vi "ApproachingPart_WangYunong.vi"() -> ()   [LabVIEW 2014]
uses:
  <vilib>/Instr/_visa.llb/VISA Configure Serial Port (Instr).vi
panel:
  in  "ZFinalHeldPos um":dbl
  out "Not Ascend of RZ":bool
  out "AfterMax":dbl
  out "RefCurr":dbl format="%#_13g"
  out "RoughZMov":dbl(graph)
  out "RZPos?":string
  out "CURR":string
  out "POS":dbl(graph)
  out "step":i32
  out "Err1":string
  in  "stop":bool
  out "Curr to Step":dbl(graph)
  out "Curr to Pos":cluster{dbl[], dbl[]}(graph)
  out "ZPos?":dbl
  out "RoughZERR?":string
  out "PIZERR?":string
  in  "ConstantCurrPIZ":refnum<visa-resource-name>="COM1"
  in  "Amp":refnum<visa-resource-name>="GPIB0::8::INSTR"
  in  "Moving":refnum<visa-resource-name>="COM6"
  out "OutLeak":string
  in  "ZApproachingThresholdDecline %":dbl format="%#_13g"
  in  "ZApproachPerStep um":dbl format="%#_13g"
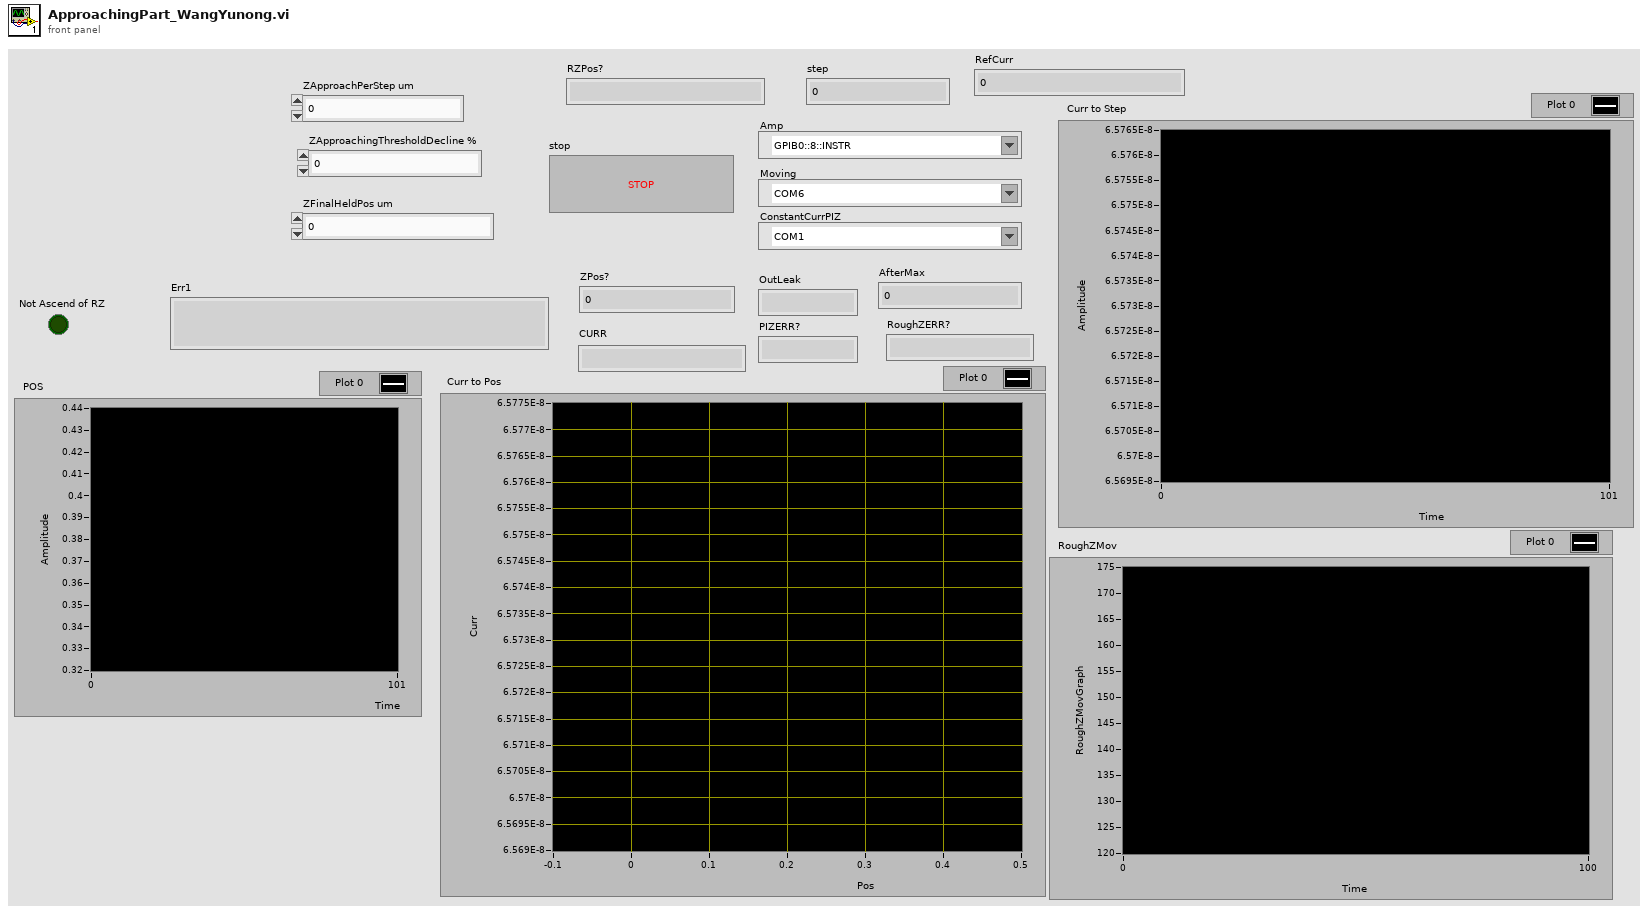
[diagram p1: front panel]
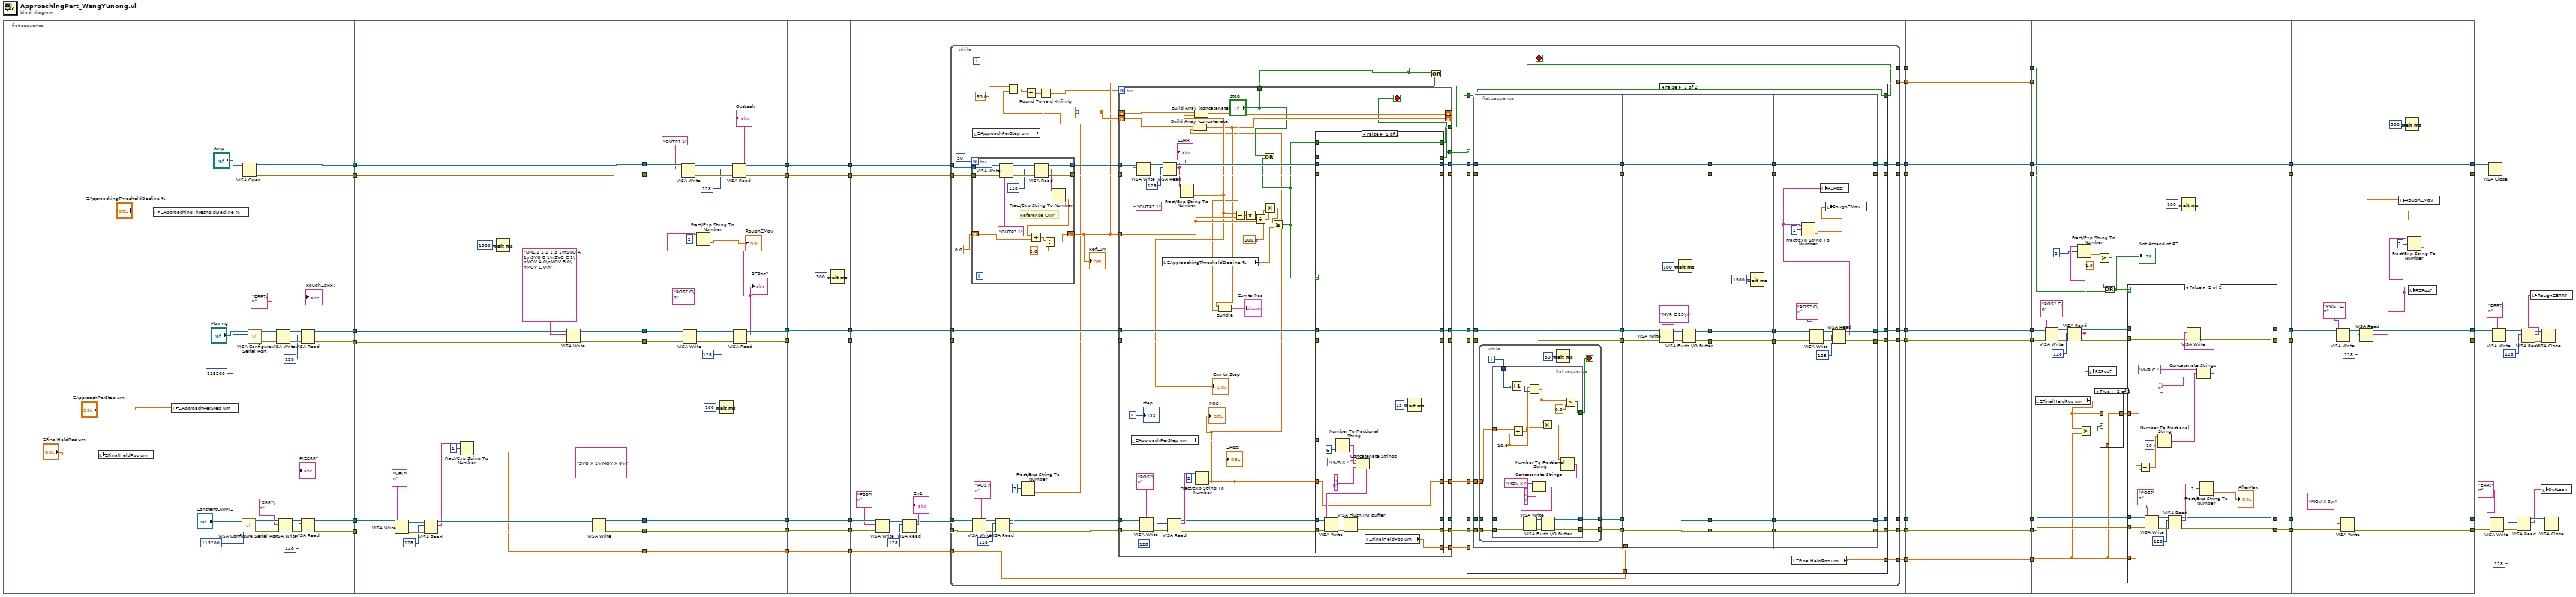
[diagram p0: block diagram]
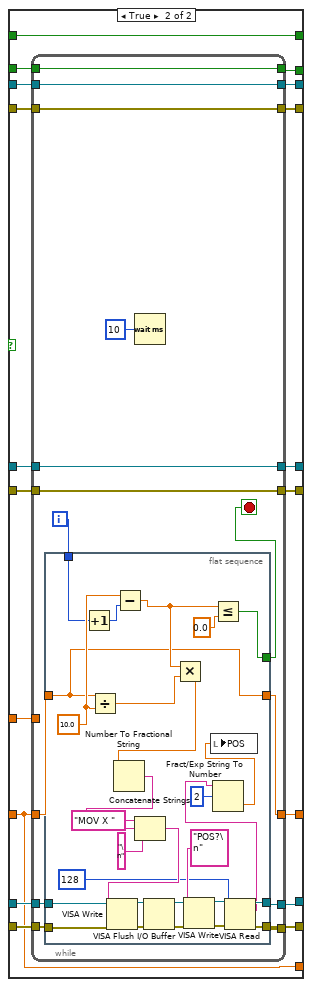
[diagram p3: hidden frame]
diagram:
  n1 = flat-sequence {
    tunnel: [w88] -> w53
    tunnel: [w87] -> w52
    tunnel: [w82] -> w51
    tunnel: [w81] -> w50
    tunnel: [w77] -> w49
    tunnel: [w76] -> w48
    tunnel: [w121] -> w71
    tunnel: [w120] -> w70
    tunnel: [w104] -> w69
    tunnel: [w103] -> w68
    tunnel: [w118] -> w67
    tunnel: [w117] -> w66
    tunnel: w53 -> [w104]
    tunnel: w52 -> [w103]
    tunnel: w51 -> [w106]
    tunnel: w50 -> [w105]
    tunnel: w49 -> [w111]
    tunnel: w48 -> [w110]
    tunnel: [w100] -> w47
    tunnel: w71 -> [w131]
    tunnel: w70 -> [w130]
    tunnel: w69 -> [w145]
    tunnel: w68 -> [w144]
    tunnel: [w129] -> w60
    tunnel: [w128] -> w61
    tunnel: [w143] -> w62
    tunnel: [w142] -> w63
    tunnel: w67 -> [w123]
    tunnel: w66 -> [w122]
    tunnel: [w123] -> w64
    tunnel: [w122] -> w65
    tunnel: w47 -> [w135]
    tunnel: [w135] -> w45
    tunnel: w65 -> [w153]
    tunnel: [w153] -> w59
    tunnel: w64 -> [w152]
    tunnel: [w152] -> w58
    tunnel: w63 -> [w151]
    tunnel: [w151] -> w57
    tunnel: w62 -> [w150]
    tunnel: [w150] -> w56
    tunnel: w61 -> [w149]
    tunnel: [w149] -> w55
    tunnel: w60 -> [w148]
    tunnel: [w148] -> w54
    tunnel: [w146] -> w46
    tunnel: w45 -> [w146]
    tunnel: w59 -> [w159]
    tunnel: w58 -> [w160]
    tunnel: w57 -> [w173]
    tunnel: w56 -> [w174]
    tunnel: w55 -> [w175]
    tunnel: w54 -> [w176]
    tunnel: [w172] -> w18
    tunnel: [w171] -> w16
    tunnel: [w170] -> w14
    tunnel: [w169] -> w12
    tunnel: [w168] -> w10
    tunnel: [w167] -> w8
    tunnel: [w166] -> w6
    tunnel: w46 -> [w165]
    tunnel: [w154] -> w4
    tunnel: [w155] -> w2
    tunnel: w18 -> [w489]
    tunnel: [w489] -> w17
    tunnel: w16 -> [w488]
    tunnel: [w488] -> w15
    tunnel: w14 -> [w487]
    tunnel: [w487] -> w13
    tunnel: w12 -> [w486]
    tunnel: [w486] -> w11
    tunnel: w10 -> [w485]
    tunnel: [w485] -> w9
    tunnel: w8 -> [w484]
    tunnel: [w484] -> w7
    tunnel: w6 -> [w483]
    tunnel: [w483] -> w5
    tunnel: w4 -> [w482]
    tunnel: [w482] -> w3
    tunnel: w2 -> [w481]
    tunnel: [w481] -> w1
    tunnel: w17 -> [w517]
    tunnel: w15 -> [w516]
    tunnel: w13 -> [w504]
    tunnel: w11 -> [w503]
    tunnel: w9 -> [w514]
    tunnel: w7 -> [w513]
    tunnel: w5 -> [_]
    tunnel: w3 -> [w490]
    tunnel: [w510] -> w44
    tunnel: [w509] -> w43
    tunnel: [w512] -> w42
    tunnel: [w511] -> w41
    tunnel: [w517] -> w40
    tunnel: [w516] -> w39
    tunnel: w1 -> [w495]
    tunnel: w44 -> [w560]
    tunnel: w43 -> [w559]
    tunnel: w42 -> [w551]
    tunnel: w41 -> [w550]
    tunnel: w40 -> [w554]
    tunnel: w39 -> [w553]
    tunnel: [w558] -> w31
    tunnel: [w557] -> w30
    tunnel: [w548] -> w27
    tunnel: [w547] -> w26
    tunnel: [w554] -> w29
    tunnel: [w553] -> w28
    frame #0 {
      n2 = local write "ZFinalHeldPos um"("ZFinalHeldPos um") -> ()
      n3 = local write "ZApproachingThresholdDecline %"("ZApproachingThresholdDecline %") -> ()
      n4 = local write "ZApproachPerStep um"("ZApproachPerStep um") -> ()
      n5 = call-poly "VISA Configure Serial Port"("VISA resource name"="ConstantCurrPIZ", "baud rate (9600)"=u32 115200) -> ("VISA resource name out"=w95:refnum<visa-resource-name>, "error out"=w94:errorcluster)  [unwired: 12 in]
      n6 = VISA Open(VISA resource name="Amp") -> (VISA resource name=w88:refnum<visa-resource-name>, error out=w87:errorcluster)  [unwired: 4 in]
      n7 = call-poly "VISA Configure Serial Port"("VISA resource name"="Moving", "baud rate (9600)"=u32 115200) -> ("VISA resource name out"=w92:refnum<visa-resource-name>, "error out"=w91:errorcluster)  [unwired: 12 in]
      n8 = VISA Write(VISA resource name=w92, write buffer="ERR?\n", error in (no error)=w91) -> (VISA resource name out=w83:refnum<visa-resource-name>, error out=w84:errorcluster)  [unwired: 1 out]
      n9 = VISA Write(VISA resource name=w95, write buffer="ERR?\n", error in (no error)=w94) -> (VISA resource name out=w79:refnum<visa-resource-name>, error out=w78:errorcluster)  [unwired: 1 out]
      n10 = VISA Read(VISA resource name=w83, byte count=u32 128, error in (no error)=w84) -> (VISA resource name out=w82:refnum<visa-resource-name>, read buffer=→"RoughZERR?":string, error out=w81:errorcluster)  [unwired: 1 out]
      n11 = VISA Read(VISA resource name=w79, byte count=u32 128, error in (no error)=w78) -> (VISA resource name out=w77:refnum<visa-resource-name>, read buffer=→"PIZERR?":string, error out=w76:errorcluster)  [unwired: 1 out]
    }
    frame #1 {
      n12 = VISA Write(VISA resource name=w111, write buffer="VEL?\n", error in (no error)=w110) -> (VISA resource name out=w114:refnum<visa-resource-name>, error out=w113:errorcluster)  [unwired: 1 out]
      n13 = VISA Read(VISA resource name=w114, byte count=u32 128, error in (no error)=w113) -> (VISA resource name out=w109:refnum<visa-resource-name>, read buffer=w102:string, error out=w108:errorcluster)  [unwired: 1 out]
      n14 = Fract/Exp String To Number(string=w102, offset=1) -> (number=w100:dbl)  [unwired: 2 in, 1 out]
      n15 = Wait (ms)(milliseconds to wait=u32 1500) -> ()  [unwired: 1 out]
      n16 = VISA Write(VISA resource name=w106, write buffer="ONL 1 1 2 1 3 1\nSVO A 1\nSVO B 1\nSVO C 1\nMOV A 0\nMOV B 0\nMOV C 0\n", error in (no error)=w105) -> (VISA resource name out=w121:refnum<visa-resource-name>, error out=w120:errorcluster)  [unwired: 1 out]
      n17 = VISA Write(VISA resource name=w109, write buffer="SVO X 1\nMOV X 0\n", error in (no error)=w108) -> (VISA resource name out=w118:refnum<visa-resource-name>, error out=w117:errorcluster)  [unwired: 1 out]
    }
    frame #2 {
      n18 = VISA Write(VISA resource name=w145, write buffer="OUTP? 1", error in (no error)=w144) -> (VISA resource name out=w141:refnum<visa-resource-name>, error out=w140:errorcluster)  [unwired: 1 out]
      n19 = VISA Write(VISA resource name=w131, write buffer="POS? C\n", error in (no error)=w130) -> (VISA resource name out=w134:refnum<visa-resource-name>, error out=w133:errorcluster)  [unwired: 1 out]
      n20 = Wait (ms)(milliseconds to wait=u32 100) -> ()  [unwired: 1 out]
      n21 = VISA Read(VISA resource name=w141, byte count=u32 128, error in (no error)=w140) -> (VISA resource name out=w143:refnum<visa-resource-name>, read buffer=→"OutLeak":string, error out=w142:errorcluster)  [unwired: 1 out]
      n22 = VISA Read(VISA resource name=w134, byte count=u32 128, error in (no error)=w133) -> (VISA resource name out=w129:refnum<visa-resource-name>, read buffer=w124:string, error out=w128:errorcluster)  [unwired: 1 out]
      "RZPos?" <- w124
      n23 = Fract/Exp String To Number(string=w124, offset=2) -> (number=→"RoughZMov":dbl)  [unwired: 2 in, 1 out]
    }
    frame #3 {
      n24 = Wait (ms)(milliseconds to wait=u32 300) -> ()  [unwired: 1 out]
    }
    frame #4 {
      n25 = VISA Write(VISA resource name=w160, write buffer="ERR?\n", error in (no error)=w159) -> (VISA resource name out=w164:refnum<visa-resource-name>, error out=w163:errorcluster)  [unwired: 1 out]
      n26 = VISA Read(VISA resource name=w164, byte count=u32 128, error in (no error)=w163) -> (VISA resource name out=w158:refnum<visa-resource-name>, read buffer=→"Err1":string, error out=w157:errorcluster)  [unwired: 1 out]
      n27 = while {
        tunnel: w176 -> [w218]
        tunnel: w175 -> [w216]
        tunnel: w174 -> [w223]
        tunnel: w173 -> [w222]
        tunnel: w158 -> [w186]
        tunnel: w157 -> [w185]
        tunnel: [w210] -> w170
        tunnel: [w209] -> w169
        tunnel: [w208] -> w172
        tunnel: [w207] -> w171
        tunnel: [w206] -> w168
        tunnel: [w205] -> w167
        tunnel: [w200] -> w166
        tunnel: w165 -> [w204]
        tunnel: [w198] -> w155
        tunnel: [w197] -> w154
        stop <- w194 stop-if-true
        w203 = dbl[] []
        n28 = for {
          N: 50 -> [_]
          tunnel: w223 -> [w232]
          tunnel: w222 -> [w231]
          tunnel: [w230] -> w220
          tunnel: [w229] -> w219
          shift-right: [w224] -> w200
          shift-left: 0.0 -> [w227]
          # "Reference Curr"
          n29 = VISA Write(VISA resource name=w232, write buffer="OUTP? 1", error in (no error)=w231) -> (VISA resource name out=w237:refnum<visa-resource-name>, error out=w236:errorcluster)  [unwired: 1 out]
          n30 = VISA Read(VISA resource name=w237, byte count=u32 128, error in (no error)=w236) -> (VISA resource name out=w230:refnum<visa-resource-name>, read buffer=w233:string, error out=w229:errorcluster)  [unwired: 1 out]
          n31 = Fract/Exp String To Number(string=w233) -> (number=w228:dbl)  [unwired: 3 in, 1 out]
          n32 = Add(x=w228, y=w227) -> (x+y=w226:dbl)
          n33 = Divide(x=w226, y=2.0) -> (x/y=w224:dbl)
        }
        "RefCurr" <- w200
        n34 = local read "ZApproachPerStep um"() -> (w178:dbl)
        n35 = VISA Write(VISA resource name=w186, write buffer="POS?\n", error in (no error)=w185) -> (VISA resource name out=w192:refnum<visa-resource-name>, error out=w191:errorcluster)  [unwired: 1 out]
        n36 = VISA Read(VISA resource name=w192, byte count=u32 128, error in (no error)=w191) -> (VISA resource name out=w184:refnum<visa-resource-name>, read buffer=w188:string, error out=w183:errorcluster)  [unwired: 1 out]
        n37 = Fract/Exp String To Number(string=w188, offset=2) -> (number=w177:dbl)  [unwired: 2 in, 1 out]
        n38 = Subtract(x=30.0, y=w177) -> (x-y=w181:dbl)
        n39 = Divide(x=w181, y=w178) -> (x/y=w180:dbl)
        n40 = Round Toward -Infinity(1:w180) -> (0:w179:dbl)
        n41 = for {
          N: w179 -> [_]
          tunnel: w184 -> [w377]
          tunnel: w183 -> [w376]
          tunnel: w200 -> [w391]
          tunnel: w220 -> [w395]
          tunnel: w219 -> [w394]
          tunnel: [w387] -> w212
          tunnel: [w386] -> w211
          tunnel: w218 -> [w385]
          tunnel: [w384] -> w217
          tunnel: w216 -> [w383]
          tunnel: [w382] -> w215
          tunnel: [w380] -> w214
          tunnel: [w379] -> w213
          tunnel: [w378] -> w202
          tunnel: [w369] -> w199
          shift-right: [w365] -> _
          shift-left: w203 -> [w368]
          shift-right: [w364] -> _
          shift-left: w203 -> [w367]
          tunnel: ["stop"] -> w198
          tunnel: [w351] -> w196
          tunnel: [w350] -> w193
          i -> [w358]
          stop <- w350 stop-if-true
          n42 = local read "ZApproachPerStep um"() -> (w381:dbl)
          n43 = VISA Write(VISA resource name=w395, write buffer="OUTP? 1", error in (no error)=w394) -> (VISA resource name out=w398:refnum<visa-resource-name>, error out=w397:errorcluster)  [unwired: 1 out]
          n44 = VISA Write(VISA resource name=w377, write buffer="POS?\n", error in (no error)=w376) -> (VISA resource name out=w375:refnum<visa-resource-name>, error out=w374:errorcluster)  [unwired: 1 out]
          n45 = local read "ZApproachingThresholdDecline %"() -> (w390:dbl)
          n46 = VISA Read(VISA resource name=w398, byte count=u32 128, error in (no error)=w397) -> (VISA resource name out=w389:refnum<visa-resource-name>, read buffer=w352:string, error out=w388:errorcluster)  [unwired: 1 out]
          "CURR" <- w352
          n47 = VISA Read(VISA resource name=w375, byte count=u32 128, error in (no error)=w374) -> (VISA resource name out=w360:refnum<visa-resource-name>, read buffer=w371:string, error out=w359:errorcluster)  [unwired: 1 out]
          n48 = Fract/Exp String To Number(string=w352) -> (number=w366:dbl)  [unwired: 3 in, 1 out]
          "Curr to Step" <- w366
          n49 = Build Array (concatenate)(w368, w366) -> (w365:dbl[])
          n50 = Fract/Exp String To Number(string=w371, offset=2) -> (number=w357:dbl)  [unwired: 2 in, 1 out]
          "ZPos?" <- w357
          "POS" <- w357
          n51 = Build Array (concatenate)(w367, w357) -> (w364:dbl[])
          n52 = Bundle(w364, w365) -> (→"Curr to Pos":cluster{dbl[], dbl[]})  [unwired: 1 in]
          n53 = Subtract(x=w366, y=w391) -> (x-y=w393:dbl)
          n54 = Absolute Value(x=w393) -> (abs(x)=w392:dbl)
          n55 = Divide(x=w392, y=w391) -> (x/y=w356:dbl)
          n56 = Multiply(x=w356, y=100.0) -> (x*y=w354:dbl)
          n57 = Greater Or Equal?(x=w354, y=w390) -> (x >= y?=w361:bool)
          n58 = Or(x="stop", y=w361) -> (x .or. y?=w353:bool)
          n59 = case shown="False" w361 {
            tunnel: w389 -> [w420 w431]
            tunnel: w388 -> [w419 w429]
            tunnel: [w420 w432] -> w387
            tunnel: [w419 w430] -> w386
            tunnel: w385 -> [w418 w427]
            tunnel: [w418 w428] -> w384
            tunnel: w383 -> [w417 w425]
            tunnel: [w417 w426] -> w382
            tunnel: w360 -> [w416 w437]
            tunnel: w359 -> [w415 w436]
            tunnel: w381 -> [w406 w433]
            tunnel: [w410 w435] -> w380
            tunnel: [w409 w434] -> w379
            tunnel: [w403 w438] -> w378
            tunnel: w361 -> [w403 w438]
            tunnel: w357 -> [w402 w421]
            tunnel: [w402 w424] -> w369
            tunnel: w353 -> [w401 w423]
            tunnel: [w401 w422] -> w350
            tunnel: [w400 w421] -> w351
            frame False {
              n60 = Number To Fractional String(number=w406, precision (6)=i16 6) -> (F-format string=w414:string)  [unwired: 2 in]
              n61 = Concatenate Strings("MVR X ", w414, "\n") -> (w411:string)
              n62 = VISA Write(VISA resource name=w416, write buffer=w411, error in (no error)=w415) -> (VISA resource name out=w408:refnum<visa-resource-name>, error out=w407:errorcluster)  [unwired: 1 out]
              n63 = VISA Flush I/O Buffer(VISA resource name=w408, error in (no error)=w407) -> (VISA resource name out=w410:refnum<visa-resource-name>, error out=w409:errorcluster)  [unwired: 1 in]
              n64 = local read "ZFinalHeldPos um"() -> (w400:dbl)
              n65 = Wait (ms)(milliseconds to wait=u32 15) -> ()  [unwired: 1 out]
            }
            frame True {
              n66 = while {
                tunnel: w437 -> [w446]
                tunnel: w436 -> [w445]
                tunnel: w421 -> [w444]
                tunnel: [w448] -> w435
                tunnel: [w447] -> w434
                tunnel: w433 -> [_]
                tunnel: [w452] -> w432
                tunnel: w431 -> [w452]
                tunnel: [w451] -> w430
                tunnel: w429 -> [w451]
                tunnel: [w450] -> w428
                tunnel: w427 -> [w450]
                tunnel: [w449] -> w426
                tunnel: w425 -> [w449]
                tunnel: [w441] -> w424
                tunnel: w423 -> [w439]
                tunnel: [w439] -> w422
                i -> [w443]
                stop <- w442 stop-if-true
                n67 = flat-sequence {
                  tunnel: w443 -> [w458]
                  tunnel: w446 -> [w478]
                  tunnel: w445 -> [w477]
                  tunnel: [w467] -> w448
                  tunnel: [w466] -> w447
                  tunnel: [w461] -> w442
                  tunnel: w444 -> [w455]
                  tunnel: [w455] -> w441
                  frame #0 {
                    w460 = 10.0
                    n68 = Increment(x=w458) -> (x+1=w459:i32)
                    n69 = Divide(x=w455, y=w460) -> (x/y=w454:dbl)
                    n70 = Subtract(x=w460, y=w459) -> (x-y=w456:dbl)
                    n71 = Multiply(x=w456, y=w454) -> (x*y=w453:dbl)
                    n72 = Number To Fractional String(number=w453) -> (F-format string=w476:string)  [unwired: 3 in]
                    n73 = Concatenate Strings("MOV X " ("string"), w476, "\n" ("string")) -> (w473:string)
                    n74 = VISA Write(VISA resource name=w478, write buffer=w473, error in (no error)=w477) -> (VISA resource name out=w480:refnum<visa-resource-name>, error out=w479:errorcluster)  [unwired: 1 out]
                    n75 = VISA Flush I/O Buffer(VISA resource name=w480, error in (no error)=w479) -> (VISA resource name out=w472:refnum<visa-resource-name>, error out=w471:errorcluster)  [unwired: 1 in]
                    n76 = VISA Write(VISA resource name=w472, write buffer="POS?\n", error in (no error)=w471) -> (VISA resource name out=w469:refnum<visa-resource-name>, error out=w468:errorcluster)  [unwired: 1 out]
                    n77 = Less Or Equal?(x=w456, y=0.0) -> (x <= y?=w461:bool)
                    n78 = VISA Read(VISA resource name=w469, byte count=u32 128, error in (no error)=w468) -> (VISA resource name out=w467:refnum<visa-resource-name>, read buffer=w463:string, error out=w466:errorcluster)  [unwired: 1 out]
                    n79 = Fract/Exp String To Number(string=w463, offset=2) -> (number=w462:dbl)  [unwired: 2 in, 1 out]
                    n80 = local write "POS"(w462) -> ()
                  }
                }
                n81 = Wait (ms)(milliseconds to wait=u32 10) -> ()  [unwired: 1 out]
              }
            }
          }
          "step" <- w358
        }
        n82 = Or(x=w198, y=w202) -> (x .or. y?=w195:bool)
        n83 = case shown="False" w193 {
          tunnel: w217 -> [w267 w349]
          tunnel: w215 -> [w266 w348]
          tunnel: w214 -> [w265 w345]
          tunnel: w213 -> [w264 w344]
          tunnel: w212 -> [w271 w347]
          tunnel: w211 -> [w269 w346]
          tunnel: [w263 w349] -> w210
          tunnel: [w262 w348] -> w209
          tunnel: [w270 w347] -> w208
          tunnel: [w268 w346] -> w207
          tunnel: [w261 w345] -> w206
          tunnel: [w260 w344] -> w205
          tunnel: w204 -> [w259 _]
          tunnel: w199 -> [w240 _]
          tunnel: [w238 w343] -> w197
          tunnel: w196 -> [_ w343]
          tunnel: w195 -> [w239 w342]
          tunnel: [w239 w342] -> w194
          frame False {
            n84 = flat-sequence {
              tunnel: w271 -> [w277]
              tunnel: w269 -> [w278]
              tunnel: w267 -> [w279]
              tunnel: w266 -> [w280]
              tunnel: w265 -> [w276]
              tunnel: w264 -> [w275]
              tunnel: [w273] -> w246
              tunnel: [w274] -> w245
              tunnel: [w280] -> w244
              tunnel: [w279] -> w243
              tunnel: [w278] -> w242
              tunnel: [w277] -> w241
              tunnel: w240 -> [w272]
              tunnel: [w319] -> w258
              tunnel: [w318] -> w256
              tunnel: [w310] -> w254
              tunnel: [w309] -> w252
              tunnel: [w312] -> w250
              tunnel: [w311] -> w248
              tunnel: w259 -> [_]
              tunnel: w246 -> [w309]
              tunnel: w245 -> [w310]
              tunnel: w244 -> [w314]
              tunnel: w243 -> [w315]
              tunnel: w242 -> [w318]
              tunnel: w241 -> [w319]
              tunnel: w258 -> [w326]
              tunnel: [w326] -> w257
              tunnel: w256 -> [w325]
              tunnel: [w325] -> w255
              tunnel: w254 -> [w324]
              tunnel: [w324] -> w253
              tunnel: w252 -> [w323]
              tunnel: [w323] -> w251
              tunnel: w250 -> [w322]
              tunnel: [w322] -> w249
              tunnel: w248 -> [w321]
              tunnel: [w321] -> w247
              tunnel: [w340] -> w268
              tunnel: [w341] -> w270
              tunnel: w257 -> [w341]
              tunnel: w255 -> [w340]
              tunnel: w253 -> [w339]
              tunnel: w251 -> [w338]
              tunnel: w249 -> [w333]
              tunnel: w247 -> [w332]
              tunnel: [w331] -> w263
              tunnel: [w330] -> w262
              tunnel: [w339] -> w261
              tunnel: [w338] -> w260
              frame #0 {
                n85 = while {
                  tunnel: w276 -> [w288]
                  tunnel: w275 -> [w287]
                  tunnel: [w286] -> w274
                  tunnel: [w285] -> w273
                  tunnel: w272 -> [w282]
                  i -> [w284]
                  stop <- w283 stop-if-true
                  n86 = flat-sequence {
                    tunnel: w284 -> [w297]
                    tunnel: w288 -> [w305]
                    tunnel: w287 -> [w304]
                    tunnel: [w303] -> w286
                    tunnel: [w302] -> w285
                    tunnel: [w290] -> w283
                    tunnel: w282 -> [w295]
                    frame #0 {
                      w294 = 10.0 ("y")
                      n87 = Increment(x=w297) -> (x+1=w296:i32)
                      n88 = Divide(x=w295, y=w294) -> (x/y=w293:dbl)
                      n89 = Subtract(x=w294, y=w296) -> (x-y=w291:dbl)
                      n90 = Multiply(x=w291, y=w293) -> (x*y=w289:dbl)
                      n91 = Number To Fractional String(number=w289) -> (F-format string=w301:string)  [unwired: 3 in]
                      n92 = Concatenate Strings("MOV X " ("string"), w301, "\n" ("string")) -> (w298:string)
                      n93 = VISA Write(VISA resource name=w305, write buffer=w298, error in (no error)=w304) -> (VISA resource name out=w307:refnum<visa-resource-name>, error out=w306:errorcluster)  [unwired: 1 out]
                      n94 = VISA Flush I/O Buffer(VISA resource name=w307, error in (no error)=w306) -> (VISA resource name out=w303:refnum<visa-resource-name>, error out=w302:errorcluster)  [unwired: 1 in]
                      n95 = Less Or Equal?(x=w291, y=0.0) -> (x <= y?=w290:bool)
                    }
                  }
                  n96 = Wait (ms)(milliseconds to wait=u32 30) -> ()  [unwired: 1 out]
                }
              }
              frame #1 {
                n97 = VISA Write(VISA resource name=w315, write buffer="MVR C 25\n", error in (no error)=w314) -> (VISA resource name out=w317:refnum<visa-resource-name>, error out=w316:errorcluster)  [unwired: 1 out]
                n98 = Wait (ms)(milliseconds to wait=u32 100) -> ()  [unwired: 1 out]
                n99 = VISA Flush I/O Buffer(VISA resource name=w317, error in (no error)=w316) -> (VISA resource name out=w312:refnum<visa-resource-name>, error out=w311:errorcluster)  [unwired: 1 in]
              }
              frame #2 {
                n100 = Wait (ms)(milliseconds to wait=u32 1500) -> ()  [unwired: 1 out]
              }
              frame #3 {
                n101 = VISA Write(VISA resource name=w333, write buffer="POS? C\n", error in (no error)=w332) -> (VISA resource name out=w336:refnum<visa-resource-name>, error out=w335:errorcluster)  [unwired: 1 out]
                n102 = VISA Read(VISA resource name=w336, byte count=u32 128, error in (no error)=w335) -> (VISA resource name out=w331:refnum<visa-resource-name>, read buffer=w329:string, error out=w330:errorcluster)  [unwired: 1 out]
                n103 = Fract/Exp String To Number(string=w329, offset=2) -> (number=w327:dbl)  [unwired: 2 in, 1 out]
                n104 = local write "RZPos?"(w329) -> ()
                n105 = local write "RoughZMov"(w327) -> ()
              }
            }
            n106 = local read "ZFinalHeldPos um"() -> (w238:dbl)
          }
          frame True {
          }
        }
      }
    }
    frame #5 {
    }
    frame #6 {
      n107 = local read "ZFinalHeldPos um"() -> (w492:dbl)
      n108 = VISA Write(VISA resource name=w504, write buffer="POS? C\n", error in (no error)=w503) -> (VISA resource name out=w507:refnum<visa-resource-name>, error out=w506:errorcluster)  [unwired: 1 out]
      n109 = VISA Read(VISA resource name=w507, byte count=u32 128, error in (no error)=w506) -> (VISA resource name out=w502:refnum<visa-resource-name>, read buffer=w500:string, error out=w501:errorcluster)  [unwired: 1 out]
      n110 = Fract/Exp String To Number(string=w500, offset=2) -> (number=w498:dbl)  [unwired: 2 in, 1 out]
      n111 = Greater?(x=w492, y=w490) -> (0:w493:bool)
      n112 = local write "RZPos?"(w500) -> ()
      n113 = Greater?(x=w498, y=1.0) -> (0:w496:bool)
      n114 = case shown="True" w493 {
        tunnel: w492 -> [w518 _]
        tunnel: [w518 w519] -> w491
        tunnel: w490 -> [_ w519]
        frame False {
        }
        frame True {
        }
      }
      n115 = Or(x=w496, y=w495) -> (x .or. y?=w494:bool)
      "Not Ascend of RZ" <- w494
      n116 = case shown="False" w494 {
        tunnel: w502 -> [w523 w526]
        tunnel: w501 -> [w522 w525]
        tunnel: w514 -> [w521 w534]
        tunnel: w513 -> [w520 w533]
        tunnel: w490 -> [_ w532]
        tunnel: [w521 w531] -> w512
        tunnel: [w520 w530] -> w511
        tunnel: [w523 w529] -> w510
        tunnel: [w522 w528] -> w509
        tunnel: w491 -> [_ w524]
        frame True {
        }
        frame False {
          n117 = Subtract(x=w532, y=w524) -> (x-y=w545:dbl)
          n118 = VISA Write(VISA resource name=w534, write buffer="POS?\n", error in (no error)=w533) -> (VISA resource name out=w539:refnum<visa-resource-name>, error out=w538:errorcluster)  [unwired: 1 out]
          n119 = Number To Fractional String(number=w545, precision (6)=i16 10) -> (F-format string=w543:string)  [unwired: 2 in]
          n120 = VISA Read(VISA resource name=w539, byte count=u32 128, error in (no error)=w538) -> (VISA resource name out=w531:refnum<visa-resource-name>, read buffer=w536:string, error out=w530:errorcluster)  [unwired: 1 out]
          n121 = Concatenate Strings("MVR C " ("string"), w543, "\n" ("F-format string")) -> (w546:string)
          n122 = VISA Write(VISA resource name=w526, write buffer=w546, error in (no error)=w525) -> (VISA resource name out=w529:refnum<visa-resource-name>, error out=w528:errorcluster)  [unwired: 1 out]
          n123 = Fract/Exp String To Number(string=w536, offset=2) -> (number=→"AfterMax":dbl)  [unwired: 2 in, 1 out]
        }
      }
      n124 = Wait (ms)(milliseconds to wait=u32 100) -> ()  [unwired: 1 out]
    }
    frame #7 {
      n125 = VISA Write(VISA resource name=w560, write buffer="POS? C\n", error in (no error)=w559) -> (VISA resource name out=w564:refnum<visa-resource-name>, error out=w563:errorcluster)  [unwired: 1 out]
      n126 = VISA Write(VISA resource name=w551, write buffer="MOV X 0\n", error in (no error)=w550) -> (VISA resource name out=w548:refnum<visa-resource-name>, error out=w547:errorcluster)  [unwired: 1 out]
      n127 = VISA Read(VISA resource name=w564, byte count=u32 128, error in (no error)=w563) -> (VISA resource name out=w558:refnum<visa-resource-name>, read buffer=w556:string, error out=w557:errorcluster)  [unwired: 1 out]
      n128 = Wait (ms)(milliseconds to wait=u32 500) -> ()  [unwired: 1 out]
      n129 = Fract/Exp String To Number(string=w556, offset=2) -> (number=w555:dbl)  [unwired: 2 in, 1 out]
      n130 = local write "RoughZMov"(w555) -> ()
      n131 = local write "RZPos?"(w556) -> ()
    }
  }
  n132 = VISA Close(VISA resource name=w29, error in (no error)=w28) -> ()  [unwired: 1 out]
  n133 = VISA Write(VISA resource name=w27, write buffer="ERR?\n", error in (no error)=w26) -> (VISA resource name out=w25:refnum<visa-resource-name>, error out=w24:errorcluster)  [unwired: 1 out]
  n134 = VISA Write(VISA resource name=w31, write buffer="ERR?\n", error in (no error)=w30) -> (VISA resource name out=w35:refnum<visa-resource-name>, error out=w34:errorcluster)  [unwired: 1 out]
  n135 = VISA Read(VISA resource name=w25, byte count=u32 128, error in (no error)=w24) -> (VISA resource name out=w23:refnum<visa-resource-name>, read buffer=w19:string, error out=w22:errorcluster)  [unwired: 1 out]
  n136 = VISA Read(VISA resource name=w35, byte count=u32 128, error in (no error)=w34) -> (VISA resource name out=w37:refnum<visa-resource-name>, read buffer=w32:string, error out=w36:errorcluster)  [unwired: 1 out]
  n137 = local write "RoughZERR?"(w32) -> ()
  n138 = local write "OutLeak"(w19) -> ()
  n139 = VISA Close(VISA resource name=w37, error in (no error)=w36) -> ()  [unwired: 1 out]
  n140 = VISA Close(VISA resource name=w23, error in (no error)=w22) -> ()  [unwired: 1 out]
